vi "Auto BAP4B.vi"(8 "mode set":T3, 10 "system state in":T1) -> (2 "system state out":T1)   [LabVIEW 2014]
doc: "Auto BAP4B\n\nSets the lights on for the Automatic State according to the mode. Transitions between \"go's,\" \"cautions.\"and \"turns\" and updates the system state based off of time remaining and change state.\n\nBeverly Abadines\nPHY 350\nP4"
uses:
  typedefs/control mode enum.ctl
  typedefs/system state cluster.ctl
  typedefs/state enum.ctl
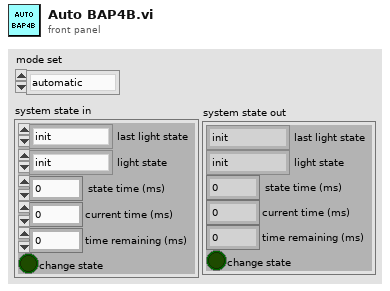
[diagram p1: front panel]
types:
  T1 = typedef "system state cluster.ctl" = cluster{"last light state":T2, "light state":T2, "state time (ms)":i32, "current time (ms)":i32, "time remaining (ms)":i32, "change state":bool}
  T2 = typedef "state enum.ctl" = enum16{"init", "idle", "left turn E", "go EW", "caution EW", "left turn W", "left turn N", "go NS", "caution NS", "left turn S", "blink on", "blink off", "all on test", "exit"}
  T3 = typedef "control mode enum.ctl" = enum16{"automatic", "blinking", "all on test"}
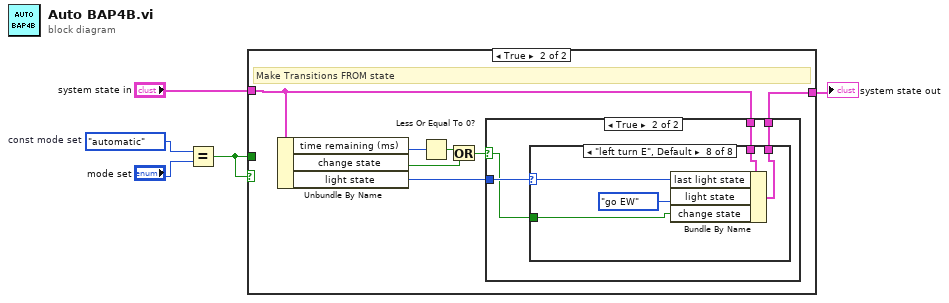
[diagram p0: block diagram]
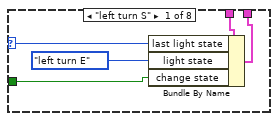
[diagram p4: hidden frame]
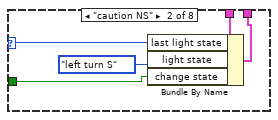
[diagram p5: hidden frame]
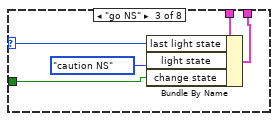
[diagram p6: hidden frame]
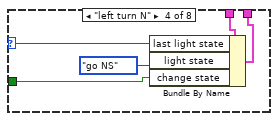
[diagram p7: hidden frame]
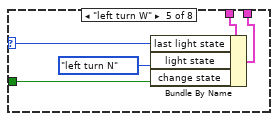
[diagram p8: hidden frame]
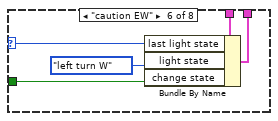
[diagram p9: hidden frame]
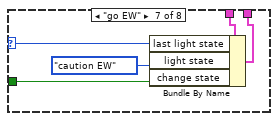
[diagram p10: hidden frame]
diagram:
  w5 = control_mode_enum."automatic"  # const mode set
  n1 = Equal?(x=w5, y="mode set") -> (x = y?=w2:bool)
  n2 = case shown="True" w2 {
    tunnel: "system state in" -> [w6 w11]
    tunnel: w2 -> [_ _]
    tunnel: [w6 w10] -> w1
    frame False {
    }
    frame True {
      # "Make Transitions FROM state"
      n3 = Unbundle By Name(w11) -> ("time remaining (ms)"=w13:i32, "change state"=w7:bool, "light state"=w12:T2)
      n4 = Less Or Equal To 0?(x=w13) -> (x <= 0?=w9:bool)
      n5 = Or(x=w9, y=w7) -> (x .or. y?=w8:bool)
      n6 = case shown="True" w8 {
        selector: w8 -> [_ w15]
        tunnel: w12 -> [_ w18]
        tunnel: w11 -> [w14 w17]
        tunnel: [w14 w16] -> w10
        frame False {
        }
        frame True {
          n7 = case shown="\"left turn E\", Default" w18 {
            selector: w18 -> [w22 w27 w32 w37 w42 w47 w52 w57]
            tunnel: w17 -> [w20 w25 w30 w35 w40 w46 w50 w55]
            tunnel: [w19 w24 w29 w34 w39 w45 w49 w54] -> w16
            tunnel: w15 -> [w21 w26 w31 w36 w41 w44 w51 w56]
            frame "left turn S" {
              n8 = Bundle By Name(cluster=w20, "last light state"=w22, "light state"=state_enum."left turn E" ("const light state"), "change state"=w21) -> (w19:T1)
            }
            frame "caution NS" {
              n9 = Bundle By Name(cluster=w25, "last light state"=w27, "light state"=state_enum."left turn S" ("const light state"), "change state"=w26) -> (w24:T1)
            }
            frame "go NS" {
              n10 = Bundle By Name(cluster=w30, "last light state"=w32, "light state"=state_enum."caution NS" ("const light state"), "change state"=w31) -> (w29:T1)
            }
            frame "left turn N" {
              n11 = Bundle By Name(cluster=w35, "last light state"=w37, "light state"=state_enum."go NS" ("const light state"), "change state"=w36) -> (w34:T1)
            }
            frame "left turn W" {
              n12 = Bundle By Name(cluster=w40, "last light state"=w42, "light state"=state_enum."left turn N" ("const light state"), "change state"=w41) -> (w39:T1)
            }
            frame "caution EW" {
              n13 = Bundle By Name(cluster=w46, "last light state"=w47, "light state"=state_enum."left turn W" ("const light state"), "change state"=w44) -> (w45:T1)
            }
            frame "go EW" {
              n14 = Bundle By Name(cluster=w50, "last light state"=w52, "light state"=state_enum."caution EW" ("const light state"), "change state"=w51) -> (w49:T1)
            }
            frame "left turn E", Default {
              n15 = Bundle By Name(cluster=w55, "last light state"=w57, "light state"=state_enum."go EW" ("const light state"), "change state"=w56) -> (w54:T1)
            }
          }
        }
      }
    }
  }
  "system state out" <- w1
